vi "IsInput.vi"(6 "error in":errorcluster, 9 "Terminal in":refnum<class "Terminal.lvclass">) -> (0 "error out":errorcluster, 2 "input":bool, 3 "Terminal out":refnum<class "Terminal.lvclass">)   [LabVIEW 2014, in "Terminal.lvclass"]
uses:
  Terminal.lvclass
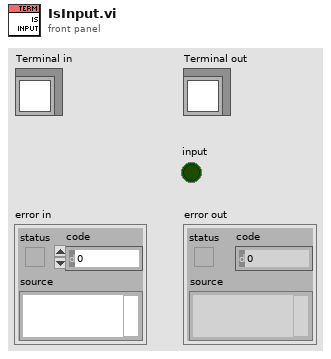
[diagram p1: front panel]
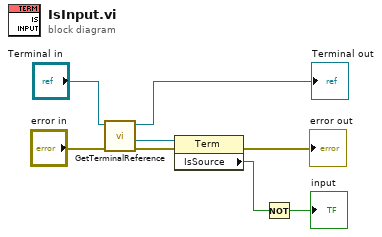
[diagram p0: block diagram]
diagram:
  n1 = call "GetTerminalReference.vi"("error in"="error in", "Terminal in"="Terminal in") -> ("error out"=w4:errorcluster, "reference"=w3:refnum<vi>, "Terminal out"=→"Terminal out":refnum<class "Terminal.lvclass">)  [unwired: 7 in]
  n2 = property class="Term"(reference=w3, error in=w4) -> (error out=→"error out":errorcluster, "IsSource"=w7:bool)  [unwired: 1 out]
  n3 = Not(x=w7) -> (.not. x?=→"input":bool)
